vi "svx_Polar_Draw_Scale.vi"(0 "picture":picture, 1 "horizontal line visible":bool=TRUE, 2 "thetaScale visible":bool=TRUE, 4 "draw rotating direct":bool, 5 "color settings":T2={"arrow color"=16860, "Magnitude major grid"=13816530, "magnitude minor grid"=16777216, "Phase grid"=13816530, "Phase scale marker text"=0}, 6 "z scale graph ref in":refnum<vi>, 7 "shaft rotating direction":u16, 8 "Polar Plot ref in":refnum<vi>, 9 "probe angle [deg]":u16, 11 "Indication Arcs":T1, 13 "Background color":u32) -> (14 "new picture":picture)   [LabVIEW 2017, in "SVX Polar Plot.xctl"]
uses:
  <vilib>/addons/_XControls/Polar Plot/SVX Polar Plot.xctl
  <vilib>/addons/_XControls/Polar Plot/subVIs/svx_Polar_Indication_Arcs.ctl
panel:
  in  "grid measurements":T3={"pixel center"={"x"=0, "y"=0}, "scale factors"={"a"=0.0, "b"=0.0, "log?(F)"=FALSE}, "grid color"=16860, "start angle"=0.0, "end angle"=360.0, "tick length"=0, "pixel radius"=0} {"end angle" format="%0.2f"; "start angle" format="%0.2f"; "scale factors"."b" format="%0.2f"; "scale factors"."a" format="%0.2f"}
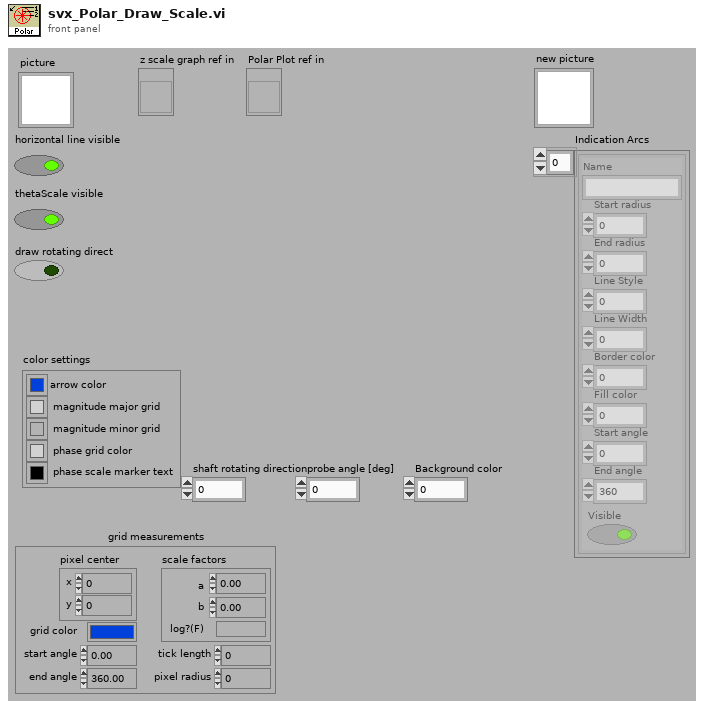
[diagram p1: front panel]
types:
  T1 = typedef "SVX Polar Plot.xctl/svx_Polar_Indication_Arcs.ctl" = cluster{"Name":string, "Start radius":dbl, "End radius":dbl, "Line Style":i32, "Line Width":i32, "Border color":u32, "Fill color":u32, "Start angle":i16, "End angle":i16, "Visible":bool}[]
  T2 = cluster{"arrow color":u32, "Magnitude major grid":u32, "magnitude minor grid":u32, "Phase grid":u32, "Phase scale marker text":u32}
  T3 = cluster{"pixel center":cluster{"x":i16, "y":i16}, "scale factors":cluster{"a":dbl, "b":dbl, "log?(F)":bool}, "grid color":u32, "start angle":dbl, "end angle":dbl, "tick length":i16, "pixel radius":i32}
  T4 = typedef "LVBoundsTypeDef.ctl" = cluster{"Width":u32, "Height":u32}
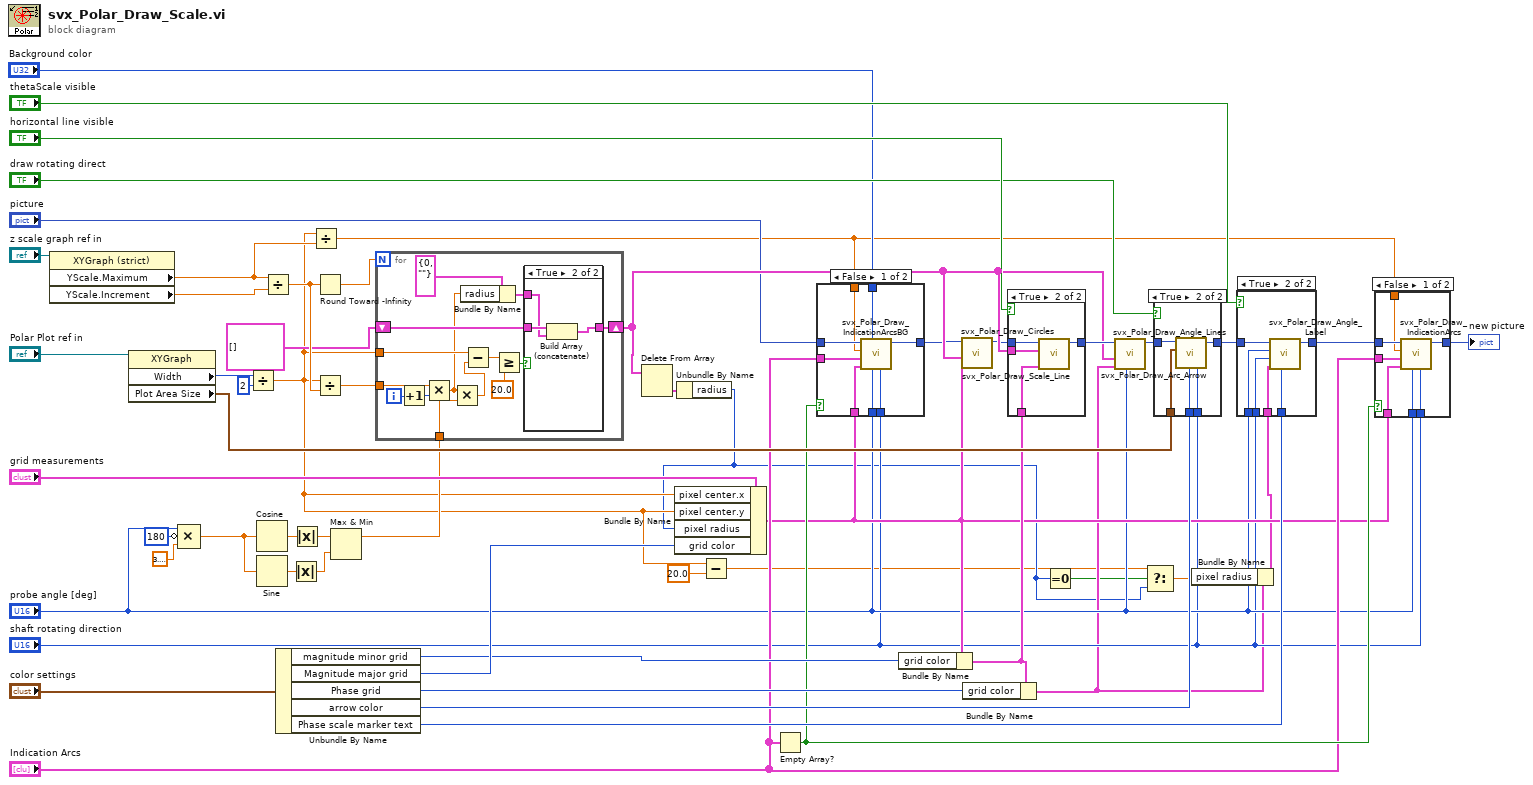
[diagram p0: block diagram]
diagram:
  n1 = property class="XYGraph (strict)"(reference="z scale graph ref in") -> ("YScale.Maximum"=w21:dbl, "YScale.Increment"=w28:dbl)  [unwired: 1 in, 2 out]
  n2 = property class="XYGraph"(reference="Polar Plot ref in") -> ("Width"=w36:u32, "Plot Area Size"=w53:T4)  [unwired: 1 in, 2 out]
  n3 = Compound Arithmetic op=MULTIPLY("probe angle [deg]", invert u16 180 ("value"), 3.141592653589793) -> (w27:dbl)
  n4 = Divide(x=w36, y=u32 2) -> (x/y=w6:dbl)
  n5 = Cosine(x=w27) -> (cos(x)=w26:dbl)
  n6 = Sine(x=w27) -> (sin(x)=w25:dbl)
  n7 = Divide(x=w21, y=w28) -> (x/y=w43:dbl)
  n8 = Unbundle By Name("color settings") -> ("magnitude minor grid"=w38:u32, "Magnitude major grid"=w47:u32, "Phase grid"=w46:u32, "arrow color"=w45:u32, "Phase scale marker text"=w48:u32)
  n9 = Absolute Value(x=w25) -> (abs(x)=w23:dbl)
  n10 = Absolute Value(x=w26) -> (abs(x)=w24:dbl)
  n11 = Divide(x=w6, y=w21) -> (x/y=w12:dbl)
  n12 = Round Toward -Infinity(1:w43) -> (0:w35:dbl)
  n13 = Divide(x=w6, y=w43) -> (x/y=w37:dbl)
  n14 = Max & Min(x=w24, y=w23) -> (max(x,y)=w22:dbl)  [unwired: 1 out]
  n15 = for {
    N: w35 -> [_]
    tunnel: w37 -> [w66]
    tunnel: w6 -> [w65]
    shift-right: [w60] -> w33
    shift-left: cluster{"radius":i16, "label":string}[] [] -> [w61]
    tunnel: w22 -> [w57]
    i -> [w68]
    n16 = Increment(x=w68) -> (x+1=w67:i32)
    n17 = Multiply(x=w66, y=w67) -> (x*y=w58:dbl)
    n18 = Multiply(x=w58, y=w57) -> (x*y=w56:dbl)
    n19 = Bundle By Name(cluster=cluster{"radius":i16, "label":string} {"radius"=0, "label"=""} ("decade specs"), "radius"=w58) -> (w62:cluster{"radius":i16, "label":string})
    n20 = Subtract(x=w65, y=w56) -> (x-y=w64:dbl)
    n21 = Greater Or Equal?(x=w64, y=20.0) -> (x >= y?=w63:bool)
    n22 = case shown="True" w63 {
      tunnel: w62 -> [_ w72]
      tunnel: w61 -> [w70 w73]
      tunnel: [w70 w71] -> w60
      frame False {
      }
      frame True {
        n23 = Build Array (concatenate)(w73, w72) -> (w71:cluster{"radius":i16, "label":string}[])
      }
    }
  }
  n24 = Delete From Array(array=w33) -> (deleted portion=w32:cluster{"radius":i16, "label":string})  [unwired: 2 in, 1 out]
  n25 = Unbundle By Name(w32) -> ("radius"=w3:i16)
  n26 = Bundle By Name(cluster="grid measurements", "pixel center.x"=w6, "pixel center.y"=w6, "pixel radius"=w3, "grid color"=w47) -> (w11:T3)
  n27 = Subtract(x=w6, y=20.0) -> (x-y=w2:dbl)
  n28 = Empty Array?(array="Indication Arcs") -> (empty?=w17:bool)
  n29 = case shown="False" w17 {
    tunnel: [w80 w82] -> w16
    tunnel: "picture" -> [w81 w82]
    tunnel: "Background color" -> [w79 _]
    tunnel: "Indication Arcs" -> [w78 _]
    tunnel: w12 -> [w77 _]
    tunnel: w11 -> [w76 _]
    tunnel: "probe angle [deg]" -> [w75 _]
    tunnel: "shaft rotating direction" -> [w74 _]
    frame False {
      n30 = call <vilib>:"svx_Polar_Draw_IndicationArcsBG.vi"("shaft rotating direction"=w74, "probe angle [deg]"=w75, "Background color"=w79, "grid measurements"=w76, "Indication Arcs"=w78, "width/max"=w77, "Picture"=w81) -> ("new picture"=w80:picture)  [unwired: 4 in]
    }
    frame True {
    }
  }
  n31 = Bundle By Name(cluster=w11, "grid color"=w38) -> (w39:T3)
  n32 = call <vilib>:"svx_Polar_Draw_Circles.vi"("grid measurements"=w11, "decade specs"=w33, "picture"=w16) -> ("new picture"=w19:picture)  [unwired: 8 in]
  n33 = Bundle By Name(cluster=w39, "grid color"=w46) -> (w8:T3)
  n34 = case shown="True" "horizontal line visible" {
    tunnel: w19 -> [w83 w87]
    tunnel: [w83 w86] -> w42
    tunnel: w33 -> [_ w85]
    tunnel: w39 -> [_ w84]
    frame False {
    }
    frame True {
      n35 = call <vilib>:"svx_Polar_Draw_Scale_Line.vi"("grid measurements"=w84, "decade specs"=w85, "picture"=w87) -> ("new picture"=w86:picture)  [unwired: 8 in]
    }
  }
  n36 = Equal To 0?(x=w3) -> (x = 0?=w4:bool)
  n37 = call <vilib>:"svx_Polar_Draw_Angle_Lines.vi"("probe angle [deg]"="probe angle [deg]", "grid measurements"=w8, "decade specs"=w33, "picture"=w42) -> ("new picture"=w50:picture)  [unwired: 7 in]
  n38 = Select(t=w2, s=w4, f=w3) -> (s? t:f=w1:dbl)
  n39 = case shown="True" "draw rotating direct" {
    tunnel: w53 -> [_ w91]
    tunnel: [w88 w92] -> w52
    tunnel: w50 -> [w88 w93]
    tunnel: w45 -> [_ w90]
    tunnel: "shaft rotating direction" -> [_ w89]
    frame False {
    }
    frame True {
      n40 = call <vilib>:"svx_Polar_Draw_Arc_Arrow.vi"("shaft rotating direction"=w89, "color"=w90, "Bounds"=w91, "Picture in"=w93) -> ("new picture"=w92:picture)  [unwired: 6 in, 1 out]
    }
  }
  n41 = Bundle By Name(cluster=w8, "pixel radius"=w1) -> (w7:T3)
  n42 = case shown="True" "thetaScale visible" {
    tunnel: w52 -> [w94 w95]
    tunnel: [w94 w100] -> w20
    tunnel: w7 -> [_ w99]
    tunnel: w48 -> [_ w98]
    tunnel: "shaft rotating direction" -> [_ w97]
    tunnel: "probe angle [deg]" -> [_ w96]
    frame False {
    }
    frame True {
      n43 = call <vilib>:"svx_Polar_Draw_Angle_Label.vi"("text color(black)"=w98, "grid measurements"=w99, "shaft rotating direction"=w97, "probe position"=w96, "Picture"=w95) -> ("new picture"=w100:picture)  [unwired: 6 in]
    }
  }
  n44 = case shown="False" w17 {
    tunnel: w20 -> [w107 w108]
    tunnel: [w106 w108] -> w18
    tunnel: "Indication Arcs" -> [w105 _]
    tunnel: w11 -> [w104 _]
    tunnel: "shaft rotating direction" -> [w103 _]
    tunnel: "probe angle [deg]" -> [w102 _]
    tunnel: w12 -> [w101 _]
    frame False {
      n45 = call <vilib>:"svx_Polar_Draw_IndicationArcs.vi"("shaft rotating direction"=w103, "probe angle [deg]"=w102, "grid measurements"=w104, "Indication Arcs"=w105, "width/max"=w101, "Picture"=w107) -> ("new picture"=w106:picture)  [unwired: 5 in]
    }
    frame True {
    }
  }
  "new picture" <- w18
